vi "Determine Change List per Section.vi"(8 "error in (no error)":errorcluster, 9 "Database Changes":T1 {"Missing"."Node Ref" format="%.0x"; "Changed"."Old"."Node Ref" format="%.0x"}, 10 "Section":string, 11 "TreeControl in":refnum<vi>) -> (0 "error out":errorcluster, 2 "Incoming":T9 {"Frames to Update"."Node Ref" format="%.0x"; "Frames to Delete" format="%.0x"}, 3 "TreeControl out":refnum<vi>)   [LabVIEW 2025, in "Protection and Counter Addon System Explorer.lvlib"]
uses:
  Protection and Counter Addon System Explorer.lvlib
  Types/VS Update List.ctl
  <vilib>/NI VeriStand/Custom Device API/Custom Device Item Ref.ctl
  Types/Base Frame Info_NoVS.ctl
  Types/Signal Attributes.ctl
  Types/CAN Filter Type.ctl
  Types/CAN Frame Update Results.ctl
  Types/Database Changes.ctl
  Types/Base Frame Info.ctl
  Types/Related CAN Frames.ctl
  Types/Related CAN Frames No VS.ctl
  <vilib>/NI VeriStand/Custom Device API/Custom Device API.lvlib
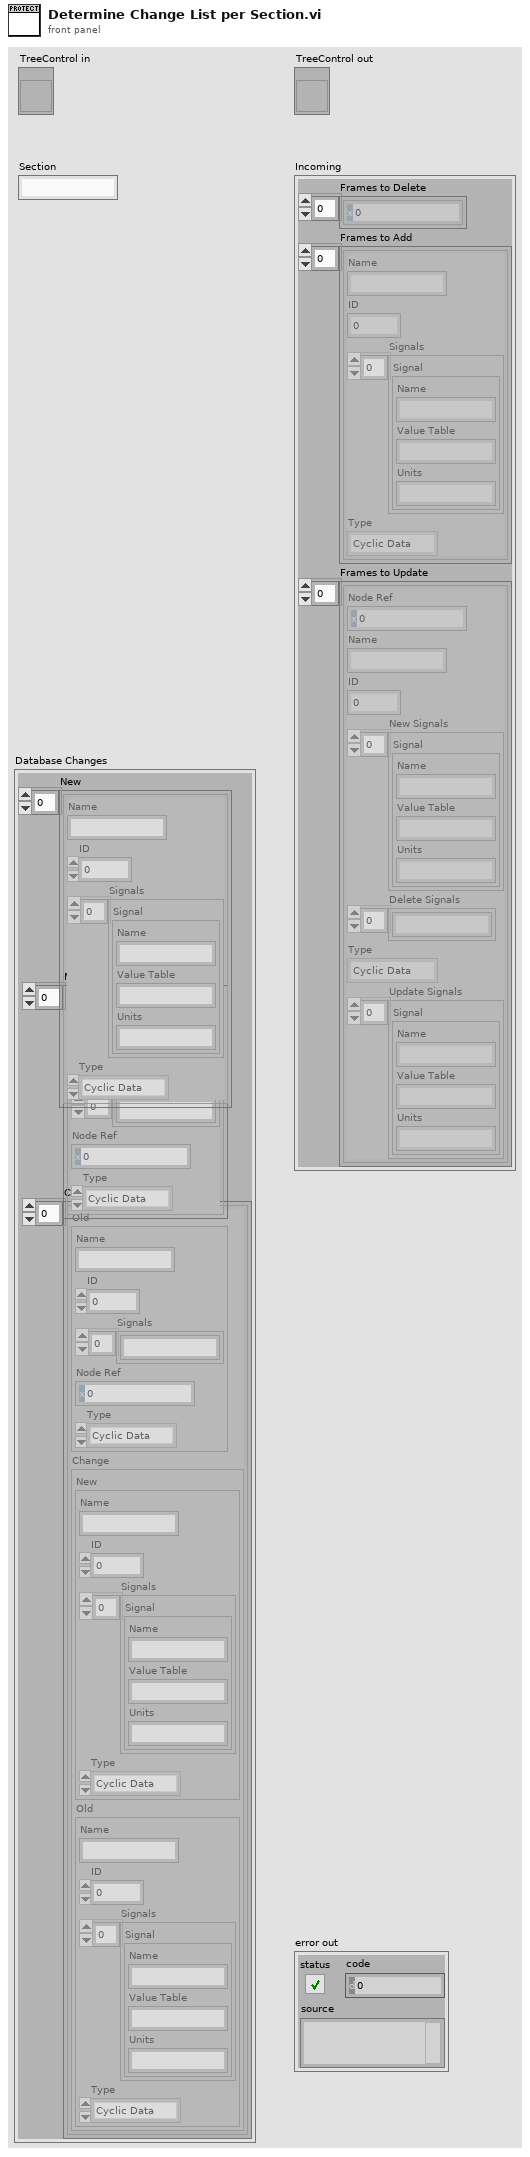
[diagram p1: front panel]
types:
  T1 = typedef "Protection and Counter Addon System Explorer.lvlib/Database Changes.ctl" = cluster{"New":T2[], "Missing":T5[], "Changed":T7[]}
  T2 = typedef "Protection and Counter Addon System Explorer.lvlib/Base Frame Info_NoVS.ctl" = cluster{"Name":string, "ID":u32, "Signals":T3[], "Type":T4}
  T3 = typedef "Protection and Counter Addon System Explorer.lvlib/Signal Attributes.ctl" = cluster{"Name":string, "Value Table":string, "Units":string}
  T4 = typedef "Protection and Counter Addon System Explorer.lvlib/CAN Filter Type.ctl" = enum16{"Cyclic Data", "Event Data", "Cyclic/Event", "All"}
  T5 = typedef "Protection and Counter Addon System Explorer.lvlib/Base Frame Info.ctl" = cluster{"Name":string, "ID":u32, "Signals":string[], "Node Ref":T6, "Type":T4}
  T6 = typedef "Custom Device API.lvlib/Custom Device Item Ref.ctl" = u64
  T7 = typedef "Protection and Counter Addon System Explorer.lvlib/Related CAN Frames.ctl" = cluster{"Old":T5, "Change":T8}
  T8 = typedef "Protection and Counter Addon System Explorer.lvlib/Related CAN Frames No VS.ctl" = cluster{"New":T2, "Old":T2}
  T9 = typedef "Protection and Counter Addon System Explorer.lvlib/VS Update List.ctl" = cluster{"Frames to Delete":T6[], "Frames to Add":T2[], "Frames to Update":T10[]}
  T10 = typedef "Protection and Counter Addon System Explorer.lvlib/CAN Frame Update Results.ctl" = cluster{"Node Ref":T6, "Name":string, "ID":u32, "New Signals":T3[], "Delete Signals":string[], "Type":T4, "Update Signals":T3[]}
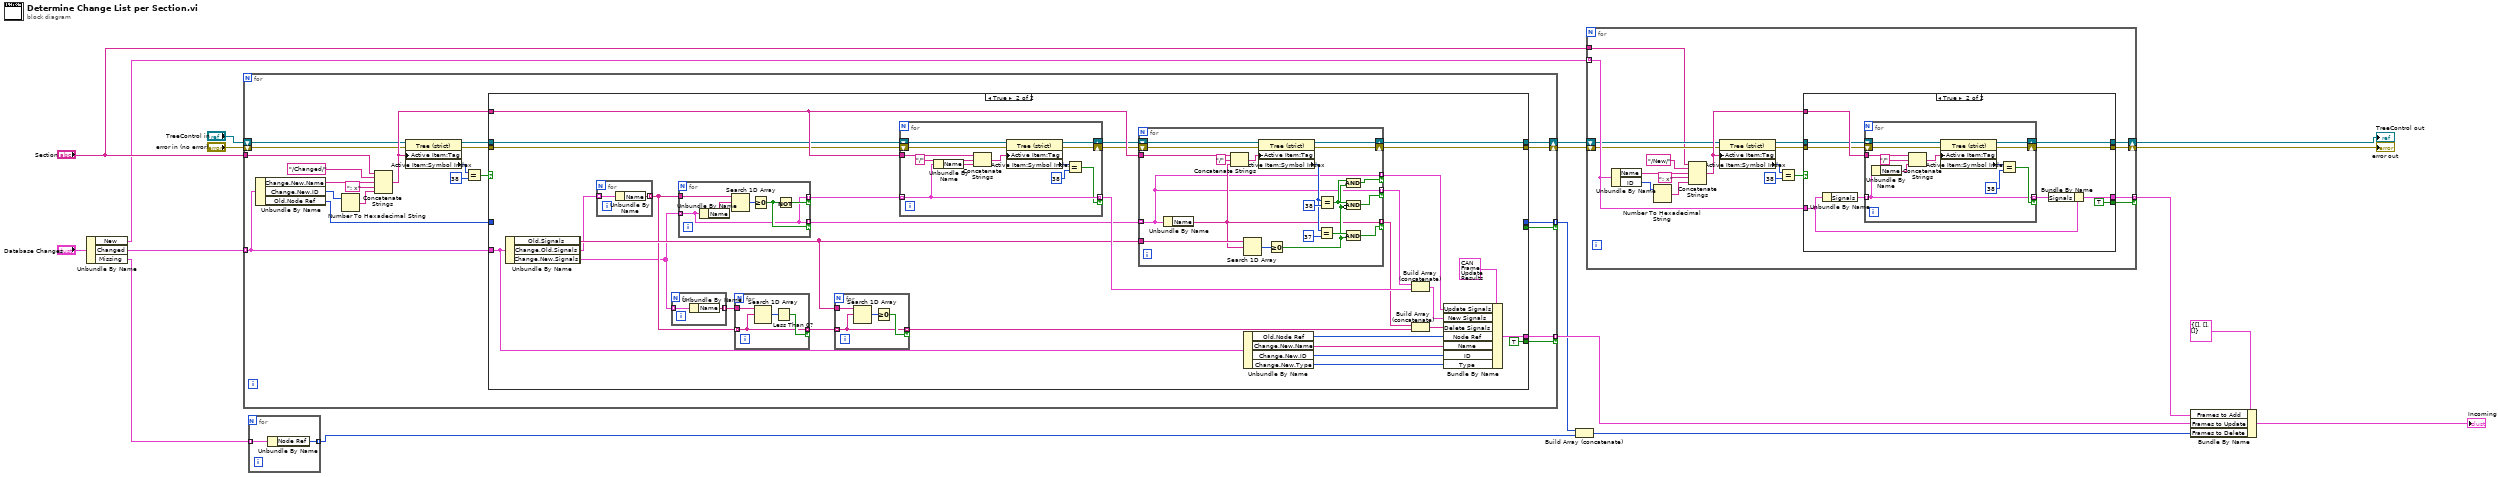
[diagram p0: block diagram]
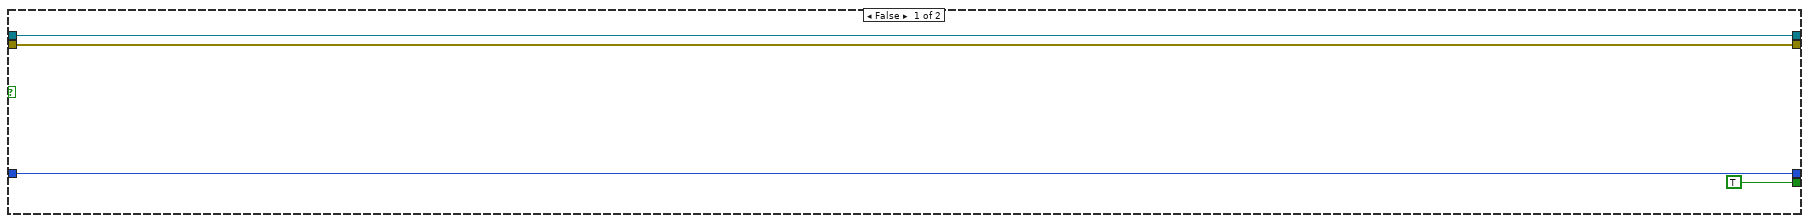
[diagram p2: hidden frame]
diagram:
  n1 = Unbundle By Name("Database Changes") -> ("New"=w8:T2[], "Changed"=w5:T7[], "Missing"=w6:T5[])
  n2 = for {
    tunnel: w5 -> [w33] mode=indexing
    tunnel: [w25] -> w1 mode=indexing if=w24
    tunnel: [w31] -> w16 mode=indexing if=w23
    shift-right: [w21] -> w9
    shift-left: "error in (no error)" -> [w28]
    shift-right: [w22] -> w11
    shift-left: "TreeControl in" -> [w27]
    tunnel: "Section" -> [w19]
    n3 = Unbundle By Name(w33) -> ("Change.New.Name"=w40:string, "Change.New.ID"=w38:u32, "Old.Node Ref"=w26:T6)
    n4 = Number To Hexadecimal String(2:w38) -> (0:w37:string)  [unwired: 1 in]
    n5 = Concatenate Strings(w19, "/Changed/" ("string"), w40, ": x" ("string"), w37) -> (w34:string)
    n6 = property class="Tree (strict)"(reference=w27, error in=w28, "Active Item:Tag"=w34) -> (reference out=w32:refnum<vi>, error out=w29:errorcluster, "Active Item:Symbol Index"=w36:i32)
    n7 = Equal?(x=w36, y=38 ("Active Item:Symbol Index")) -> (x = y?=w30:bool)
    n8 = case shown="True" w30 {
      tunnel: w34 -> [_ w71]
      tunnel: w33 -> [_ w53]
      tunnel: w32 -> [w41 w69]
      tunnel: [_ w64] -> w31
      tunnel: w26 -> [w44 _]
      tunnel: w29 -> [w42 w61]
      tunnel: [w44 _] -> w25
      tunnel: [TRUE _] -> w24
      tunnel: [_ TRUE] -> w23
      tunnel: [w41 w52] -> w22
      tunnel: [w42 w51] -> w21
      frame False {
      }
      frame True {
        n9 = Unbundle By Name(w53) -> ("Old.Signals"=w68:string[], "Change.Old.Signals"=w48:T3[], "Change.New.Signals"=w46:T3[])
        n10 = for {
          tunnel: w48 -> [w78] mode=indexing
          tunnel: [w77] -> w47 mode=indexing
          n11 = Unbundle By Name(w78) -> ("Name"=w77:string)
        }
        n12 = for {
          tunnel: w46 -> [w76] mode=indexing
          tunnel: [w75] -> w49 mode=indexing
          n13 = Unbundle By Name(w76) -> ("Name"=w75:string)
        }
        n14 = for {
          tunnel: w47 -> [w124]
          tunnel: [w119] -> w72 mode=indexing if=w122
          tunnel: [w119] -> w74 mode=indexing if=w121
          tunnel: w46 -> [w119] mode=indexing
          n15 = Unbundle By Name(w119) -> ("Name"=w120:string)
          n16 = Search 1D Array(1D array=w124, element=w120) -> (index of element=w123:i32)  [unwired: 1 in]
          n17 = Greater Or Equal To 0?(x=w123) -> (x >= 0?=w122:bool)
          n18 = Not(x=w122) -> (.not. x?=w121:bool)
        }
        n19 = for {
          tunnel: w49 -> [w118]
          tunnel: w47 -> [w115] mode=indexing
          tunnel: [w115] -> w70 mode=indexing if=w116
          n20 = Search 1D Array(1D array=w118, element=w115) -> (index of element=w117:i32)  [unwired: 1 in]
          n21 = Less Than 0?(x=w117) -> (x < 0?=w116:bool)
        }
        n22 = for {
          tunnel: w68 -> [w82]
          tunnel: w70 -> [w79] mode=indexing
          tunnel: [w79] -> w65 mode=indexing if=w80
          n23 = Search 1D Array(1D array=w82, element=w79) -> (index of element=w81:i32)  [unwired: 1 in]
          n24 = Greater Or Equal To 0?(x=w81) -> (x >= 0?=w80:bool)
        }
        n25 = for {
          tunnel: w71 -> [w112]
          tunnel: w74 -> [w110] mode=indexing
          tunnel: [w110] -> w73 mode=indexing if=w109
          shift-right: [w106] -> w63
          shift-left: w69 -> [w108]
          shift-right: [w105] -> w62
          shift-left: w61 -> [w104]
          n26 = Unbundle By Name(w110) -> ("Name"=w103:string)
          n27 = Concatenate Strings(w112, "/" ("string"), w103) -> (w107:string)
          n28 = property class="Tree (strict)"(reference=w108, error in=w104, "Active Item:Tag"=w107) -> (reference out=w106:refnum<vi>, error out=w105:errorcluster, "Active Item:Symbol Index"=w113:i32)
          n29 = Equal?(x=w113, y=38 ("Active Item:Symbol Index")) -> (x = y?=w109:bool)
        }
        n30 = for {
          tunnel: w71 -> [w101]
          tunnel: w72 -> [w84] mode=indexing
          tunnel: [w84] -> w67 mode=indexing if=w94
          tunnel: w68 -> [w96]
          tunnel: [w85] -> w66 mode=indexing if=w92
          shift-right: [w90] -> w52
          shift-left: w63 -> [w91]
          shift-right: [w88] -> w51
          shift-left: w62 -> [w89]
          tunnel: [w84] -> w45 mode=indexing if=w83
          n31 = Unbundle By Name(w84) -> ("Name"=w85:string)
          n32 = Concatenate Strings(w101, "/" ("string"), w85) -> (w99:string)
          n33 = Search 1D Array(1D array=w96, element=w85) -> (index of element=w95:i32)  [unwired: 1 in]
          n34 = property class="Tree (strict)"(reference=w91, error in=w89, "Active Item:Tag"=w99) -> (reference out=w90:refnum<vi>, error out=w88:errorcluster, "Active Item:Symbol Index"=w97:i32)
          n35 = Greater Or Equal To 0?(x=w95) -> (x >= 0?=w86:bool)
          n36 = Equal?(x=w97, y=37 ("Active Item:Symbol Index")) -> (x = y?=w93:bool)
          n37 = Equal?(x=w97, y=38 ("Active Item:Symbol Index")) -> (x = y?=w87:bool)
          n38 = Compound Arithmetic op=AND(w87, w86) -> (w83:bool)
          n39 = Compound Arithmetic op=AND(w87, invert w86) -> (w94:bool)
          n40 = Compound Arithmetic op=AND(w93, w86) -> (w92:bool)
        }
        n41 = Unbundle By Name(w53) -> ("Old.Node Ref"=w57:T6, "Change.New.Name"=w60:string, "Change.New.ID"=w56:u32, "Change.New.Type"=w50:T4)
        n42 = Build Array (concatenate)(w67, w73) -> (w55:T3[])
        n43 = Build Array (concatenate)(w66, w65) -> (w54:string[])
        n44 = Bundle By Name(cluster=T10 {"Node Ref"=0, "Name"="", "ID"=0, "New Signals"=[], "Delete Signals"=[], "Type"=enum."Cyclic Data", "Update Signals"=[]}, "Update Signals"=w45, "New Signals"=w55, "Delete Signals"=w54, "Node Ref"=w57, "Name"=w60, "ID"=w56, "Type"=w50) -> (w64:T10)
      }
    }
  }
  n45 = for {
    tunnel: w6 -> [w126] mode=indexing
    tunnel: [w125] -> w7 mode=indexing
    n46 = Unbundle By Name(w126) -> ("Node Ref"=w125:T6)
  }
  n47 = Build Array (concatenate)(w1, w7) -> (w17:T6[])
  n48 = for {
    tunnel: w8 -> [w138] mode=indexing
    tunnel: [w136] -> w15 mode=indexing if=w131
    shift-right: [w129] -> w10
    shift-left: w9 -> [w133]
    shift-right: [w130] -> w12
    shift-left: w11 -> [w132]
    tunnel: "Section" -> [w127]
    n49 = Unbundle By Name(w138) -> ("Name"=w145:string, "ID"=w143:u32)
    n50 = Number To Hexadecimal String(2:w143) -> (0:w142:string)  [unwired: 1 in]
    n51 = Concatenate Strings(w127, "/New/" ("string"), w145, ": x" ("string"), w142) -> (w139:string)
    n52 = property class="Tree (strict)"(reference=w132, error in=w133, "Active Item:Tag"=w139) -> (reference out=w137:refnum<vi>, error out=w134:errorcluster, "Active Item:Symbol Index"=w141:i32)
    n53 = Equal?(x=w141, y=38 ("Active Item:Symbol Index")) -> (x = y?=w135:bool)
    n54 = case shown="True" w135 {
      tunnel: w139 -> [_ w157]
      tunnel: w138 -> [_ w149]
      tunnel: w137 -> [w146 w156]
      tunnel: [_ w155] -> w136
      tunnel: w134 -> [w147 w154]
      tunnel: [_ TRUE] -> w131
      tunnel: [w146 w150] -> w130
      tunnel: [w147 w151] -> w129
      frame False {
      }
      frame True {
        n55 = Unbundle By Name(w149) -> ("Signals"=w152:T3[])
        n56 = for {
          tunnel: w157 -> [w167]
          tunnel: w152 -> [w158] mode=indexing
          tunnel: [w158] -> w148 mode=indexing if=w165
          shift-right: [w162] -> w150
          shift-left: w156 -> [w164]
          shift-right: [w161] -> w151
          shift-left: w154 -> [w160]
          n57 = Unbundle By Name(w158) -> ("Name"=w159:string)
          n58 = Concatenate Strings(w167, "/" ("string"), w159) -> (w163:string)
          n59 = property class="Tree (strict)"(reference=w164, error in=w160, "Active Item:Tag"=w163) -> (reference out=w162:refnum<vi>, error out=w161:errorcluster, "Active Item:Symbol Index"=w168:i32)
          n60 = Equal?(x=w168, y=38 ("Active Item:Symbol Index")) -> (x = y?=w165:bool)
        }
        n61 = Bundle By Name(cluster=w149, "Signals"=w148) -> (w155:T2)
      }
    }
  }
  "TreeControl out" <- w12
  "error out" <- w10
  n62 = Bundle By Name(cluster=T9 {"Frames to Delete"=[], "Frames to Add"=[], "Frames to Update"=[]} ("Incoming"), "Frames to Add"=w15, "Frames to Update"=w16, "Frames to Delete"=w17) -> (→"Incoming":T9)
